vi "testAppendErrorInformation_Warning_withState.vi"(8 "error in (no error)":errorcluster, 11 "testStateMachineUtilities in":refnum<class "testStateMachineUtilities.lvclass">) -> (0 "error out":errorcluster, 3 "testStateMachineUtilities out":refnum<class "testStateMachineUtilities.lvclass">)   [LabVIEW 2013, in "testStateMachineUtilities.lvclass"]
uses:
  testStateMachineUtilities.lvclass
  source/State Machine Support API/Parse State Queue_2024.vi
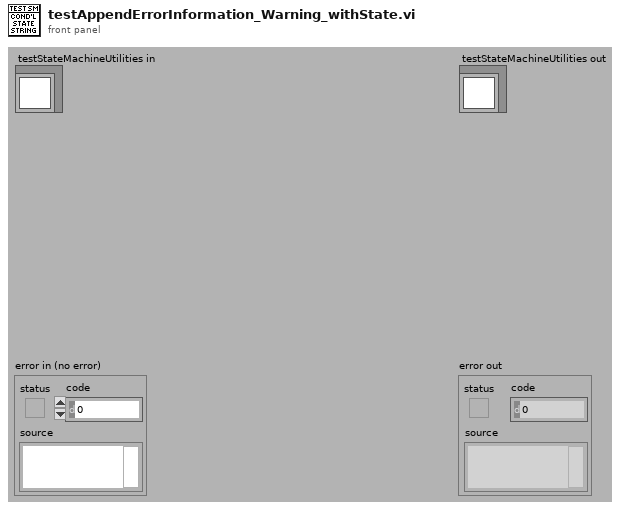
[diagram p1: front panel]
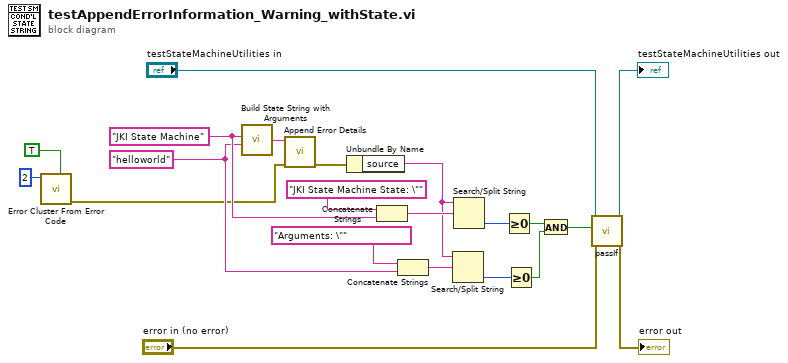
[diagram p0: block diagram]
diagram:
  w15 = "JKI State Machine" ("Previous State and Argument(s)")
  w13 = "helloworld" ("Previous State and Argument(s)")
  n1 = call <vilib>:"Error Cluster From Error Code.vi"("is warning? (False)"=TRUE, "error code (0)"=2) -> ("error out"=w5:errorcluster)  [unwired: 7 in]
  n2 = call "Build State String with Arguments.vi"("Arguments (\"\")"=w13, "State"=w15) -> ("State with Arguments"=w17:string)  [unwired: 4 in]
  n3 = call "Append Error Details.vi"("error in (no error)"=w5, "Previous State and Argument(s)"=w17) -> ("error out"=w4:errorcluster)  [unwired: 9 in]
  n4 = Unbundle By Name(w4) -> ("source"=w3:string)
  n5 = Concatenate Strings("JKI State Machine State: \"" ("search string/char (-)"), w15) -> (w10:string)
  n6 = Concatenate Strings("Arguments: \"" ("search string/char (-)"), w13) -> (w9:string)
  n7 = Search/Split String(string=w3, search string/char (-)=w9) -> (offset of match=w11:i32)  [unwired: 1 in, 2 out]
  n8 = Search/Split String(string=w3, search string/char (-)=w10) -> (offset of match=w14:i32)  [unwired: 1 in, 2 out]
  n9 = Greater Or Equal To 0?(x=w14) -> (x >= 0?=w8:bool)
  n10 = Greater Or Equal To 0?(x=w11) -> (x >= 0?=w7:bool)
  n11 = And(x=w8, y=w7) -> (x .and. y?=w2:bool)
  n12 = call-dynamic "passIf.vi"("error in (no error)"="error in (no error)", "pass"=w2, "TestCase in"="testStateMachineUtilities in") -> ("error out"=→"error out":errorcluster, "TestCase out"=→"testStateMachineUtilities out":refnum<class "testStateMachineUtilities.lvclass">)  [unwired: 7 in]
